vi "SVFA FFT Spectrum (Real-Im).vi"   [LabVIEW 2017]
doc: "Computes the Fast Fourier Transform (FFT) spectrum of <B>scaled signal [EU]</B>. This VI returns FFT results as the real and imaginary parts, or the first and second elements of the ordered pairs, of the FFT spectrum. Wire data to the <B>scaled signal [EU]</B> input to determine the polymorphic instance to use or manually select the instance."
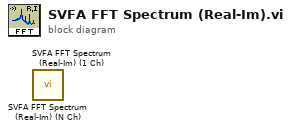
[diagram p0: block diagram]
diagram:
  n1 = call <vilib>:"SVFA FFT Spectrum (Real-Im) (N Ch).vi"() -> ()  [unwired: 13 in, 7 out]
  n2 = call <vilib>:"SVFA FFT Spectrum (Real-Im) (1 Ch).vi"() -> ()  [unwired: 13 in, 7 out]
